vi "LOC VI Tools Globals.vi"() -> ()   [LabVIEW 2020, in "Localization_Tools.lvlib"]
uses:
  Localization_Tools.lvlib
panel:
  in  "Localzation Directory":path
  in  "Mode":enum16{"Read", "Write"}(ring)
  in  "Disable Localization":bool
  in  "DebugLOC":bool
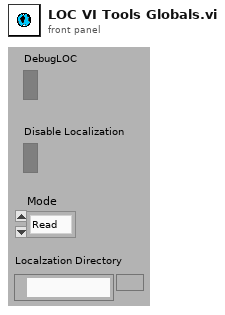
[diagram p1: front panel]
diagram:
